vi "SRS DS345 fun gen.vi"() -> ()   [LabVIEW 2014]
uses:
  <instrlib>/Stanford Research DS345/Stanford Research DS345.lvlib
panel:
  in  "Tab Control":enum32{"Manual control", "Auto control"}(tab)
  in  "Manual control":T1={"Waveform"=1, "Amplitude (V)"=3.0, "Frequency (Hz)"=1000.0} {"Frequency (Hz)" min=10.0 max=29000000.0 format="%#_8g"; "Amplitude (V)" min=0.01 max=8.0; "Waveform" items=["Sine", "Square", "Triangle", "Ramp", "Noise"]}
  in  "Auto sweep control":T2={"Waveform"=1, "Start amplitude (V)"=0.05, "Freq (Hz)"=1000.0, "End amplitude (V)"=8.0, "# of steps"=5.0, "# of scans at each ampl."=5.0} {"# of scans at each ampl." min=1.0 max=1000.0 step=1.0; "# of steps" min=1.0 max=1000.0 step=1.0; "End amplitude (V)" min=0.01 max=8.0; "Freq (Hz)" min=10.0 max=29000000.0 format="%#_8g"; "Start amplitude (V)" min=0.01 max=8.0; "Waveform" items=["Sine", "Square", "Triangle", "Ramp", "Noise"]}
  in  "begin sweep":bool
  in  "End sweep now":bool
  in  "Stop Button":bool
  # "Pulse generator"
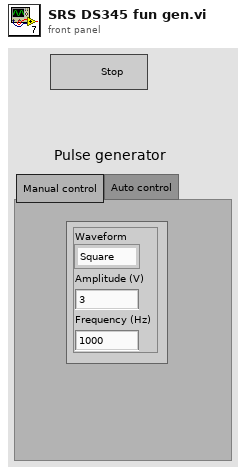
[diagram p1: front panel]
types:
  T1 = cluster{"Waveform":u16, "Amplitude (V)":dbl, "Frequency (Hz)":dbl}
  T2 = cluster{"Waveform":u16, "Start amplitude (V)":dbl, "Freq (Hz)":dbl, "End amplitude (V)":dbl, "# of steps":dbl, "# of scans at each ampl.":dbl}
  T3 = enum8{"Enabled", "Disabled", "Disabled and Grayed Out"}
  T4 = cluster{"Baud Rate":u32, "Parity":u16, "Data Bits":u16, "Stop Bits":u16, "Flow Control":u16}
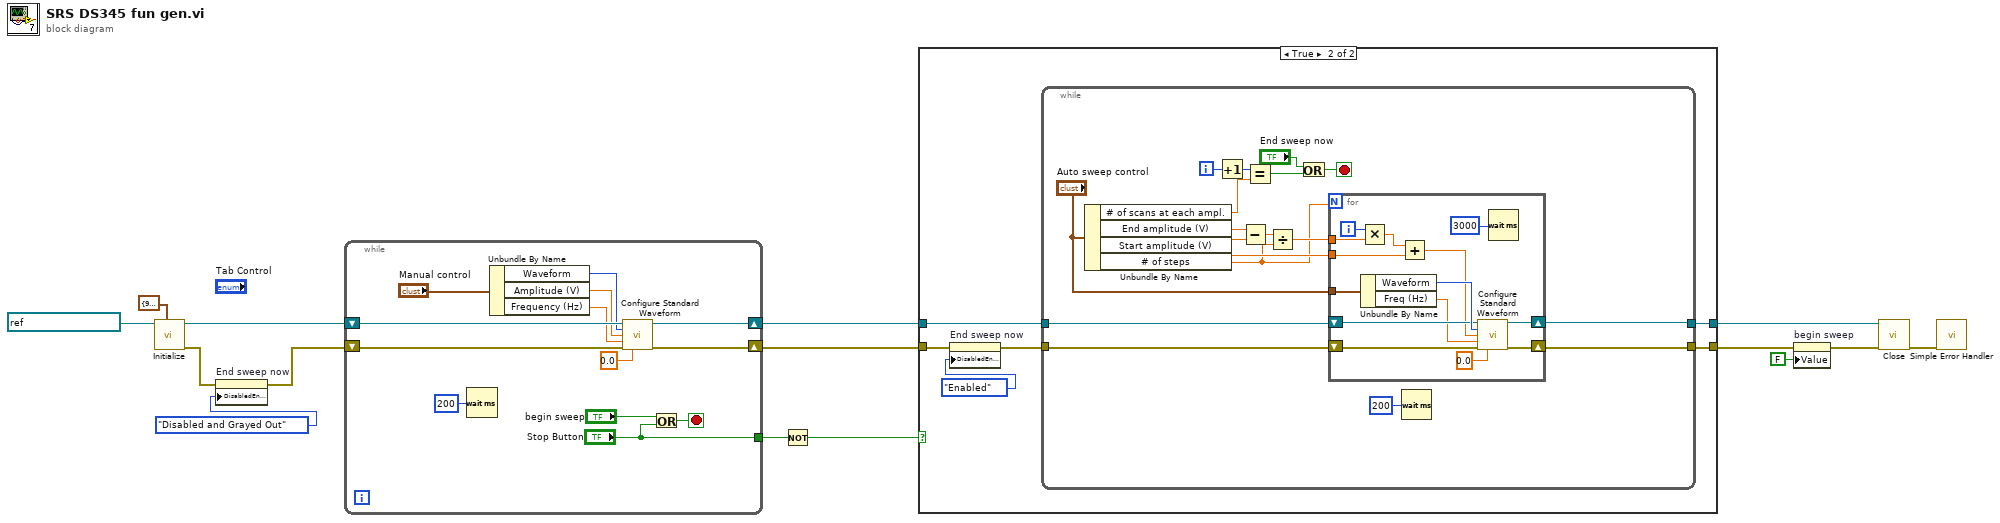
[diagram p0: block diagram]
diagram:
  n1 = call <instrlib>:"Initialize.vi"("Serial Configuration"=T4 {"Baud Rate"=9600, "Parity"=0, "Data Bits"=8, "Stop Bits"=20, "Flow Control"=0}, "VISA resource name"=refnum<visa-resource-name> "GPIB2::19::INSTR") -> ("error out"=w2:errorcluster, "VISA resource name out"=w14:refnum<visa-resource-name>)  [unwired: 8 in]
  n2 = property on="End sweep now" class="Bool"(error in=w2, "DisabledEnum"=T3."Disabled and Grayed Out" ("Disabled")) -> (error out=w1:errorcluster)  [unwired: 1 in, 1 out]
  n3 = while {
    shift-right: [w26] -> w11
    shift-left: w14 -> [w28]
    shift-right: [w25] -> w9
    shift-left: w1 -> [w27]
    tunnel: ["Stop Button"] -> w7
    stop <- w18 stop-if-true
    n4 = Wait (ms)(milliseconds to wait=u32 200) -> ()  [unwired: 1 out]
    n5 = Unbundle By Name("Manual control") -> ("Waveform"=w22:u16, "Amplitude (V)"=w21:dbl, "Frequency (Hz)"=w20:dbl)
    n6 = call <instrlib>:"Configure Standard Waveform.vi"("VISA resource name"=w28, "Waveform Function (0: Sine)"=w22, "Amplitude (0.01 Vpp)"=w21, "Frequency (1000 Hz)"=w20, "error in (no error)"=w27, "DC Offset (0.00 V)"=0.0) -> ("VISA resource name out"=w26:refnum<visa-resource-name>, "error out"=w25:errorcluster)  [unwired: 8 in]
    n7 = Or(x="begin sweep", y="Stop Button") -> (x .or. y?=w18:bool)
  }
  n8 = Not(x=w7) -> (.not. x?=w6:bool)
  n9 = case shown="True" w6 {
    tunnel: w11 -> [w30 w36]
    tunnel: [w30 w35] -> w10
    tunnel: w9 -> [w29 w32]
    tunnel: [w29 w34] -> w5
    frame False {
    }
    frame True {
      n10 = property on="End sweep now" class="Bool"(error in=w32, "DisabledEnum"=T3."Enabled" ("Disabled")) -> (error out=w31:errorcluster)  [unwired: 1 in, 1 out]
      n11 = while {
        tunnel: [w51] -> w35
        tunnel: w36 -> [w53]
        tunnel: [w50] -> w34
        tunnel: w31 -> [w52]
        i -> [w39]
        stop <- w49 stop-if-true
        n12 = Unbundle By Name("Auto sweep control") -> ("# of scans at each ampl."=w40:dbl, "End amplitude (V)"=w46:dbl, "Start amplitude (V)"=w44:dbl, "# of steps"=w43:dbl)
        n13 = Increment(x=w39) -> (x+1=w38:i32)
        n14 = Subtract(x=w46, y=w44) -> (x-y=w47:dbl)
        n15 = Equal?(x=w38, y=w40) -> (x = y?=w41:bool)
        n16 = Divide(x=w47, y=w43) -> (x/y=w45:dbl)
        n17 = Or(x="End sweep now", y=w41) -> (x .or. y?=w49:bool)
        n18 = for {
          N: w43 -> [_]
          shift-right: [w63] -> w51
          shift-left: w53 -> [w65]
          shift-right: [w62] -> w50
          shift-left: w52 -> [w64]
          tunnel: "Auto sweep control" -> [w61]
          tunnel: w45 -> [w59]
          tunnel: w44 -> [w58]
          i -> [w57]
          n19 = Multiply(x=w57, y=w59) -> (x*y=w60:dbl)
          n20 = Unbundle By Name(w61) -> ("Waveform"=w67:u16, "Freq (Hz)"=w56:dbl)
          n21 = Add(x=w60, y=w58) -> (x+y=w55:dbl)
          n22 = call <instrlib>:"Configure Standard Waveform.vi"("VISA resource name"=w65, "Waveform Function (0: Sine)"=w67, "Amplitude (0.01 Vpp)"=w55, "Frequency (1000 Hz)"=w56, "error in (no error)"=w64, "DC Offset (0.00 V)"=0.0) -> ("VISA resource name out"=w63:refnum<visa-resource-name>, "error out"=w62:errorcluster)  [unwired: 8 in]
          n23 = Wait (ms)(milliseconds to wait=u32 3000) -> ()  [unwired: 1 out]
        }
        n24 = Wait (ms)(milliseconds to wait=u32 200) -> ()  [unwired: 1 out]
      }
    }
  }
  n25 = property on="begin sweep" class="Bool (strict)"(error in=w5, "Value"=FALSE ("begin sweep")) -> (error out=w4:errorcluster)  [unwired: 1 in, 1 out]
  n26 = call <instrlib>:"Close.vi"("error in (no error)"=w4, "VISA resource name"=w10) -> ("error out"=w13:errorcluster)  [unwired: 9 in]
  n27 = call <vilib>:"Simple Error Handler.vi"("error in (no error)"=w13) -> ()  [unwired: 4 in, 5 out]
